vi "Close.vi"(8 "error in (no error)":errorcluster, 11 "HFP Gen in":refnum<class "PL HFP Generator.lvclass">) -> (0 "error out":errorcluster)   [LabVIEW 2015, in "PL HFP Generator.lvclass"]
doc: "Closes connection to device."
uses:
  PL HFP Generator.lvclass
  <vilib>/plasmapper/PL Modbus Client/PL Modbus Client.lvclass
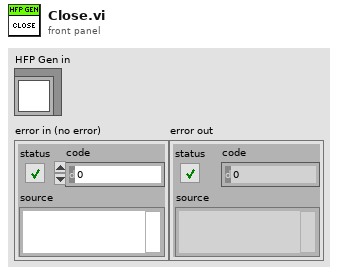
[diagram p1: front panel]
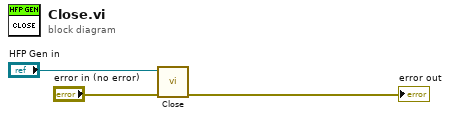
[diagram p0: block diagram]
diagram:
  n1 = call-parent "Close.vi"("error in (no error)"="error in (no error)", "MODBUS in"="HFP Gen in") -> ("error out"=→"error out":errorcluster)  [unwired: 9 in]
